vi "Product Selected.vi"(8 "error in (no error)":errorcluster, 10 "Item Sel":string[](array[string]), 11 "Controller in":refnum<class "Controller.lvclass">) -> (0 "error out":errorcluster, 3 "Controller out":refnum<class "Controller.lvclass">)   [LabVIEW 2020, in "Controller.lvlib" / "Controller.lvclass"]
uses:
  Controller.lvclass
  Controller.lvclass/Controller.ctl
  Mesage Display Messages/Update Message Msg/Update Message Msg.lvclass/Update Message Msg.ctl
  <vilib>/ActorFramework/Message Enqueuer/Message Enqueuer.lvclass/Message Enqueuer.ctl
  <vilib>/ActorFramework/Message Enqueuer/Enqueue.vi
  Mesage Display Messages/Update Message Msg/Update Message Msg.lvclass
  C:/Program Files (x86)/National Instruments/LabVIEW 2020/vi.lib/ActorFramework/Message/Message.lvclass
  <vilib>/ActorFramework/Message Priority Queue/Priority Enqueue.vi
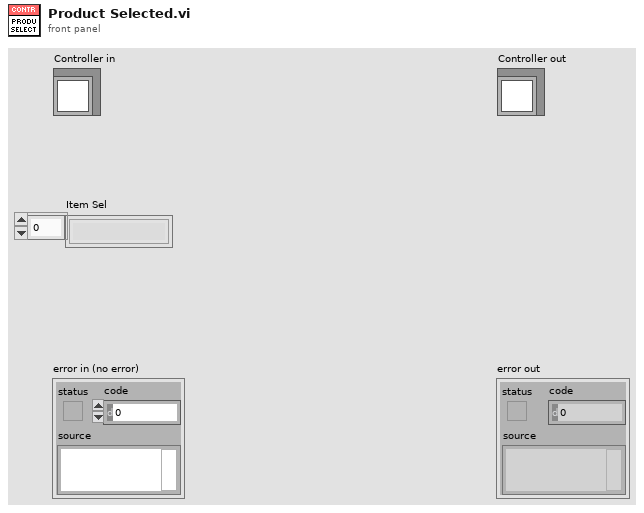
[diagram p1: front panel]
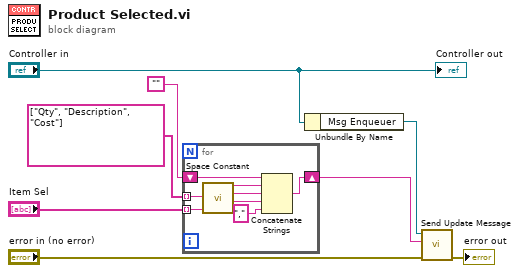
[diagram p0: block diagram]
diagram:
  n1 = for {
    tunnel: "Item Sel" -> [w12] mode=indexing
    tunnel: string[] ["Qty", "Description", "Cost"] -> [w14] mode=indexing
    shift-right: [w10] -> w3
    shift-left: "" -> [w9]
    n2 = call <vilib>:"Space Constant.vi"() -> ("String"=w13:string)
    n3 = Concatenate Strings(w9, w14, w13, w12, ",") -> (w10:string)
  }
  n4 = Unbundle By Name("Controller in") -> ("Msg Enqueuer"=w7:refnum<class "Message Enqueuer.lvclass">)
  n5 = call "Send Update Message.vi"("error in (no error)"="error in (no error)", "Msg"=w3, "Message Enqueuer"=w7) -> ("error out"=→"error out":errorcluster)  [unwired: 7 in, 1 out]
  "Controller out" <- "Controller in"
